vi "NewNYStyleVeggiePizza.vi"(8 "error in (no error)":errorcluster) -> (0 "error out":errorcluster, 3 "NYStyleVeggiePizza":refnum<class "NYStyleVeggiePizza.lvclass">)   [LabVIEW 2020, in "FactoryMethod.lvlib" / "PizzaFactoryMethod.lvlib" / "NYStyleVeggiePizza.lvclass"]
uses:
  NYStyleVeggiePizza.lvclass
  NYStyleVeggiePizza.lvclass/NYStyleVeggiePizza.ctl
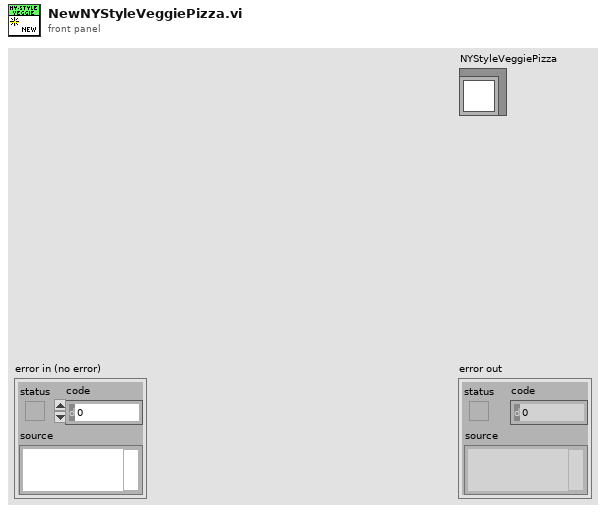
[diagram p1: front panel]
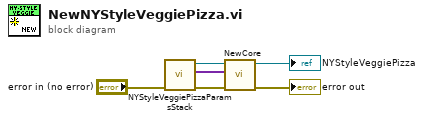
[diagram p0: block diagram]
diagram:
  n1 = call "NYStyleVeggiePizzaParamsStack.vi"("error iN"="error in (no error)") -> ("error out"=w6:errorcluster, "HierarchyParams"=w5:variant[], "NYStyleVeggiePizza"=w1:refnum<class "NYStyleVeggiePizza.lvclass">)  [unwired: 8 in]
  n2 = call-dynamic "NewCore.vi"("error in (no error)"=w6, "ParamsArray"=w5, "NYStyleVeggiePizza"=w1) -> ("error out"=→"error out":errorcluster, "NYStyleVeggiePizza"=→"NYStyleVeggiePizza":refnum<class "NYStyleVeggiePizza.lvclass">)  [unwired: 7 in]
